vi "material--AB_RW_Convert_Path_to_Relative.vi"(8 "error in":errorcluster, 10 "Theme Path":path, 11 "VI Path":path) -> (0 "error out":errorcluster, 2 "relativeType":T1, 3 "newPath":path)   [LabVIEW 2021]
doc: "adapted from @DBomm in this repo https://github.com/illuminated-g/lv-relative-paths"
uses:
  <vilib>/AppBuilder/AB_Relative_Path_Type.ctl
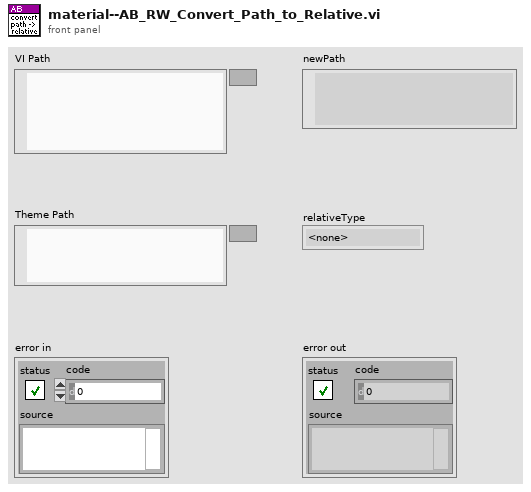
[diagram p1: front panel]
types:
  T1 = typedef "AB_Relative_Path_Type.ctl" = enum16{"<none>", "relativeToCommon", "relativeToAppDir", "relativeToProject"}
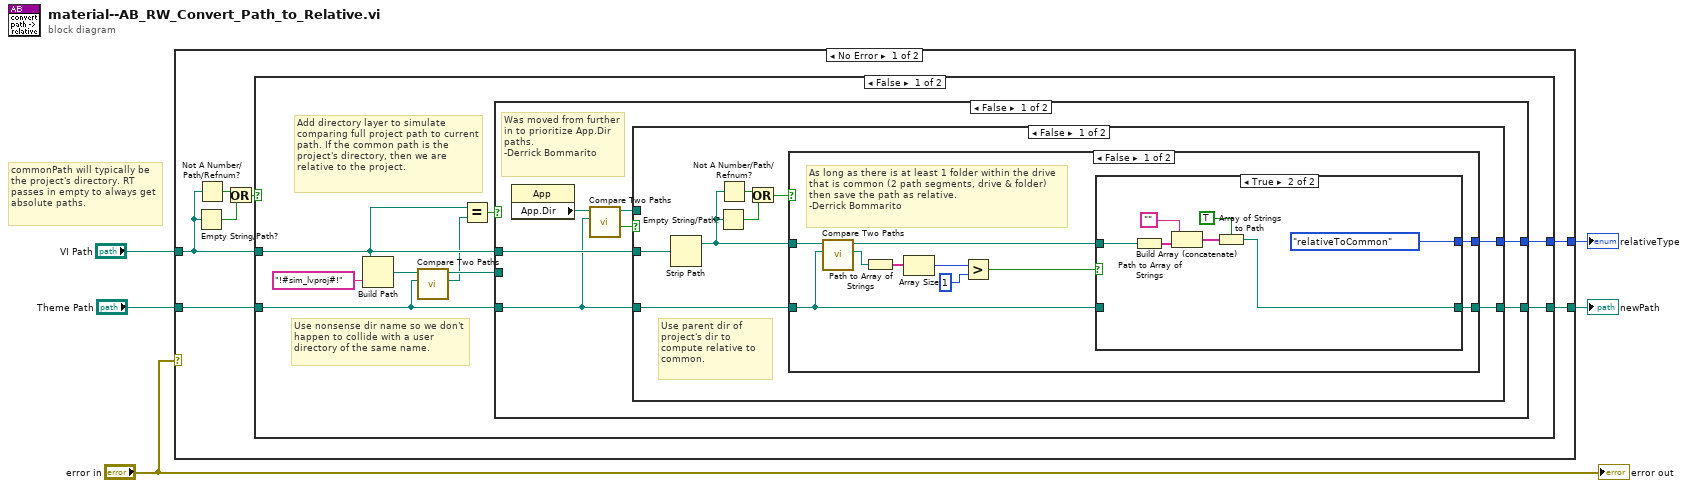
[diagram p0: block diagram]
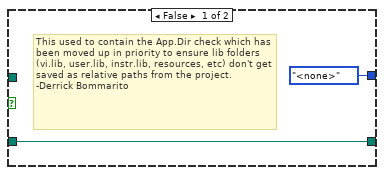
[diagram p2: hidden frame]
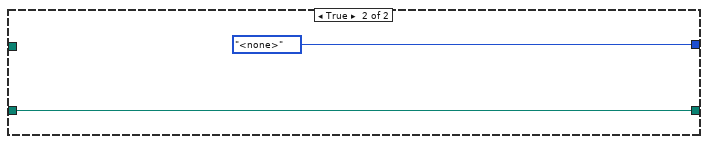
[diagram p3: hidden frame]
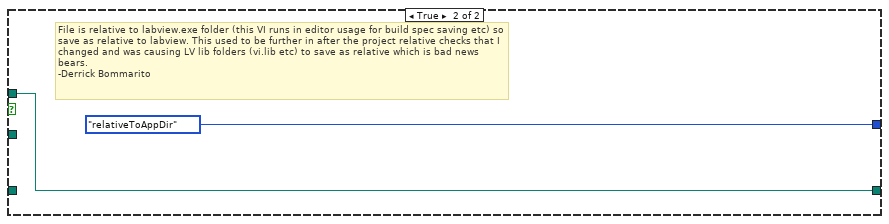
[diagram p4: hidden frame]
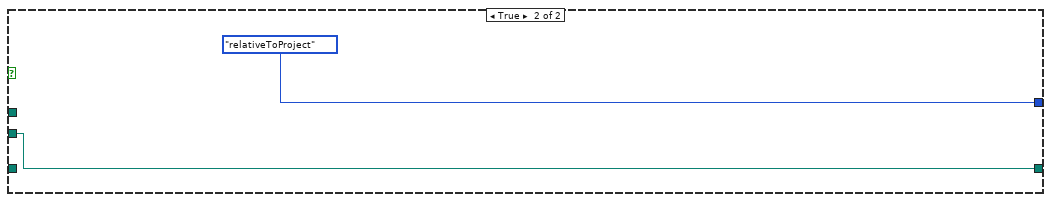
[diagram p5: hidden frame]
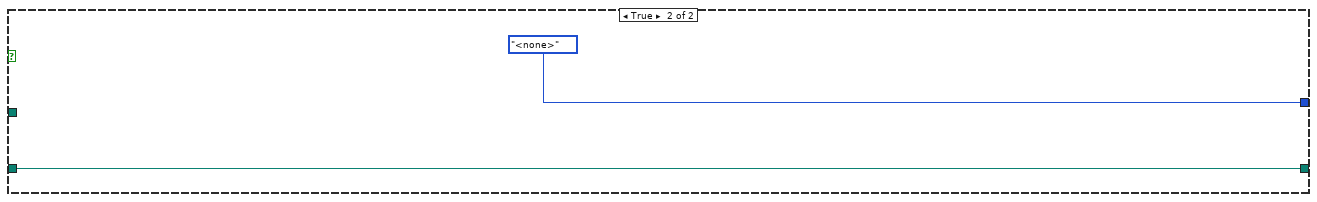
[diagram p6: hidden frame]
diagram:
  # "commonPath will typically be the project's directory. RT passes in empty to always get absolute paths."
  n1 = case shown="No Error" "error in" {
    tunnel: "VI Path" -> [w7 _]
    tunnel: "Theme Path" -> [w12 w64]
    tunnel: [w11 w64] -> w2
    tunnel: [w10 _] -> w1
    frame No Error {
      n2 = Empty String/Path?(string/path=w7) -> (empty?=w9:bool)
      n3 = Not A Number/Path/Refnum?(number/path/refnum=w7) -> (NaN/Path/Refnum?=w8:bool)
      n4 = Or(x=w8, y=w9) -> (x .or. y?=w6:bool)
      n5 = case shown="False" w6 {
        tunnel: w12 -> [w16 w63]
        tunnel: [w21 w63] -> w11
        tunnel: [w20 AB_Relative_Path_Type."<none>" ("relativeType")] -> w10
        tunnel: w7 -> [w15 _]
        frame False {
          # "Use nonsense dir name so we don't happen to collide with a user directory of the same name."
          # "Add directory layer to simulate comparing full project path to current path. If the common path is the project's directory, then we are relative to the project."
          n6 = Build Path(base path=w15, name or relative path="!#sim_lvproj#!") -> (appended path=w17:path)
          n7 = call <vilib>:"Compare Two Paths.vi"("Path 2"=w16, "Path 1"=w17) -> ("Common Path"=w14:path, "Relative Path from 1 to 2"=w18:path)  [unwired: 6 in, 2 out]
          n8 = Equal?(x=w15, y=w14) -> (x = y?=w13:bool)
          n9 = case shown="False" w13 {
            tunnel: [w28 w61] -> w21
            tunnel: [w27 AB_Relative_Path_Type."relativeToProject" ("relativeType")] -> w20
            tunnel: w15 -> [w26 _]
            tunnel: w16 -> [w24 _]
            tunnel: w18 -> [_ w61]
            frame False {
              # "Was moved from further in to prioritize App.Dir paths.\n-Derrick Bommarito"
              n10 = property class="App"() -> ("App.Dir"=w25:path)  [unwired: 2 in, 2 out]
              n11 = call <vilib>:"Compare Two Paths.vi"("Path 2"=w24, "Path 1"=w25) -> ("Path 2 Relative to Path 1?"=w23:bool, "Relative Path from 1 to 2"=w22:path)  [unwired: 6 in, 2 out]
              n12 = case shown="False" w23 {
                tunnel: [w36 w59] -> w28
                tunnel: [w35 AB_Relative_Path_Type."relativeToAppDir" ("relativeType")] -> w27
                tunnel: w26 -> [w30 _]
                tunnel: w24 -> [w29 _]
                tunnel: w22 -> [_ w59]
                frame False {
                  # "Use parent dir of project's dir to compute relative to common."
                  n13 = Strip Path(path=w30) -> (stripped path=w34:path)  [unwired: 1 out]
                  n14 = Empty String/Path?(string/path=w34) -> (empty?=w32:bool)
                  n15 = Not A Number/Path/Refnum?(number/path/refnum=w34) -> (NaN/Path/Refnum?=w33:bool)
                  n16 = Or(x=w33, y=w32) -> (x .or. y?=w31:bool)
                  n17 = case shown="False" w31 {
                    tunnel: w29 -> [w46 w57]
                    tunnel: [w45 w57] -> w36
                    tunnel: [w44 AB_Relative_Path_Type."<none>" ("relativeType")] -> w35
                    tunnel: w34 -> [w42 _]
                    frame False {
                      # "As long as there is at least 1 folder within the drive that is common (2 path segments, drive & folder) then save the path as relative.\n-Derrick Bommarito"
                      n18 = call <vilib>:"Compare Two Paths.vi"("Path 2"=w46, "Path 1"=w42) -> ("Common Path"=w41:path, "Relative Path from 1 to 2"=w43:path)  [unwired: 6 in, 2 out]
                      n19 = Path to Array of Strings(0:w41) -> (2:w40:string[])  [unwired: 1 out]
                      n20 = Array Size(array=w40) -> (size(s)=w39:i32)
                      n21 = Greater?(x=w39, y=1) -> (0:w37:bool)
                      n22 = case shown="True" w37 {
                        tunnel: w46 -> [w47 _]
                        tunnel: [w47 w49] -> w45
                        tunnel: [AB_Relative_Path_Type."<none>" ("relativeType") AB_Relative_Path_Type."relativeToCommon" ("relativeType")] -> w44
                        tunnel: w43 -> [_ w54]
                        frame False {
                          # "This used to contain the App.Dir check which has been moved up in priority to ensure lib folders (vi.lib, user.lib, instr.lib, resources, etc) don't get saved as relative paths from the project.\n-Derrick Bommarito"
                        }
                        frame True {
                          n23 = Path to Array of Strings(0:w54) -> (2:w53:string[])  [unwired: 1 out]
                          n24 = Build Array (concatenate)("", w53) -> (w51:string[])
                          n25 = Array of Strings to Path(0:w51, 1:TRUE ("relative")) -> (2:w49:path)
                        }
                      }
                    }
                    frame True {
                    }
                  }
                }
                frame True {
                  # "File is relative to labview.exe folder (this VI runs in editor usage for build spec saving etc) so save as relative to labview. This used to be further in after the project relative checks that I changed and was causing LV lib folders (vi.lib etc) to save as relative which is bad news bears.\n-Derrick Bommarito"
                }
              }
            }
            frame True {
            }
          }
        }
        frame True {
        }
      }
    }
    frame Error {
    }
  }
  "newPath" <- w2
  "relativeType" <- w1
  "error out" <- "error in"
